vi "Character Replac.vi"(11 "字符串":string) -> (3 "连接的字符串":string)   [LabVIEW 2020]
panel:
  # "Min(@功率分析仪1.CH1.MyTest01.Ims[A]@,@功率分析仪1.CH1.MyTest01.P[kW]@)*Max(@功率分析仪1.CH1.MyTest01.Vms[V]@,@功率分析仪1.CH3.Test03.P[kW]@)"
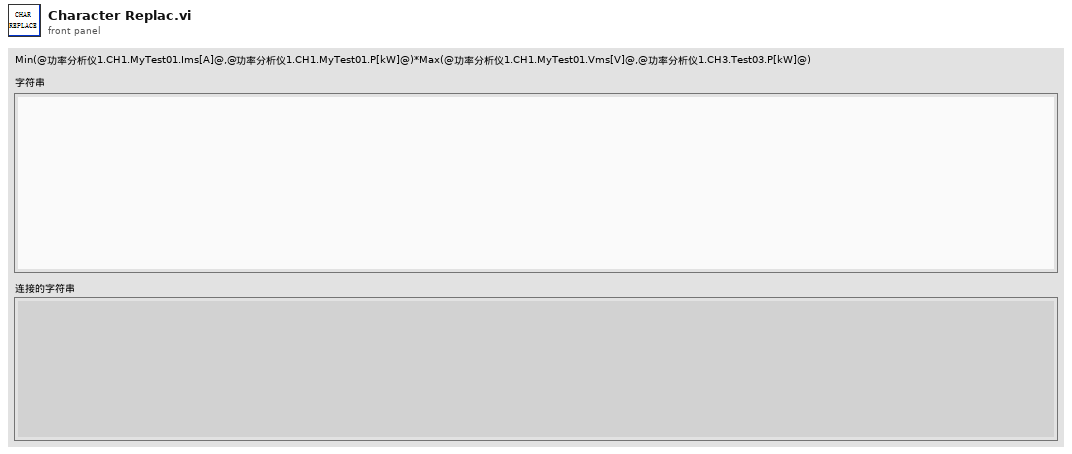
[diagram p1: front panel]
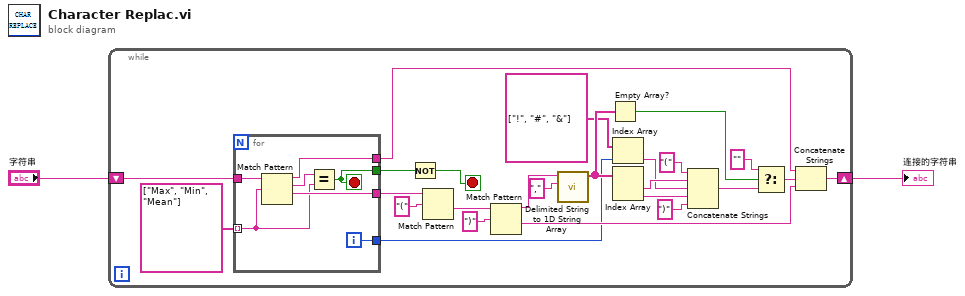
[diagram p0: block diagram]
diagram:
  n1 = while {
    shift-right: [w22] -> w2
    shift-left: "字符串" -> [w20]
    stop <- w3 stop-if-true
    n2 = for {
      tunnel: [w33] -> w19
      tunnel: string[] ["Max", "Min", "Mean"] ("搜索字符串/字符(-)") -> [w30] mode=indexing
      tunnel: w20 -> [w34]
      tunnel: [w32] -> w18
      tunnel: [w29] -> w7
      tunnel: [w28] -> w5
      i -> [w28]
      stop <- w29 stop-if-true
      n3 = Match Pattern(string=w34, regular expression=w30) -> (before substring=w32:string, match substring=w31:string, after substring=w33:string)  [unwired: 1 in, 1 out]
      n4 = Equal?(x=w31, y=w30) -> (x = y?=w29:bool)
    }
    n5 = Not(x=w7) -> (.not. x?=w3:bool)
    n6 = Match Pattern(string=w19, regular expression="(" ("搜索字符串/字符(-)")) -> (after substring=w17:string)  [unwired: 1 in, 3 out]
    n7 = Match Pattern(string=w17, regular expression=")" ("搜索字符串/字符(-)")) -> (before substring=w15:string, after substring=w14:string)  [unwired: 1 in, 2 out]
    n8 = call <vilib>:"Delimited String to 1D String Array.vi"("delimiter"=",", "delimited string"=w15) -> ("string array"=w13:string[])  [unwired: 9 in]
    n9 = Empty Array?(array=w13) -> (empty?=w12:bool)
    n10 = Index Array(array=string[] ["!", "#", "&"] ("搜索字符串/字符(-)"), index=w5) -> (element=w4:string)
    n11 = Index Array(array=w13) -> (element #1=w25:string, element #2=w21:string)  [unwired: 2 in]
    n12 = Concatenate Strings("(" ("字符串"), w25, w4, w21, ")" ("字符串")) -> (w10:string)
    n13 = Select(t="" ("连接的字符串"), s=w12, f=w10) -> (s? t:f=w9:string)
    n14 = Concatenate Strings(w18, w9, w14) -> (w22:string)
  }
  "连接的字符串" <- w2
